vi "Keithley617_IV.vi"() -> ()   [LabVIEW 2015, in "Keithley617.lvlib"]
uses:
  Keithley617.lvlib
  Keithley617_GPIB_Commands.ctl
panel:
  in  "Array":T1(array[cluster])
  out "IV- Live Plot":cluster{"X":dbl, "Y":dbl}[](graph)
  out "Error Out":errorcluster
  in  "Error In":errorcluster
  in  "GPIB Address String":string="27"
  in  "Input Parameters":T2={"Start Voltage"=0.0, "End Voltage"=0.0, "Voltage Step"=0.0, "Step Time (ms)"=100.0}
  out "IV-result":cluster{"X":dbl, "Y":dbl}[](graph)
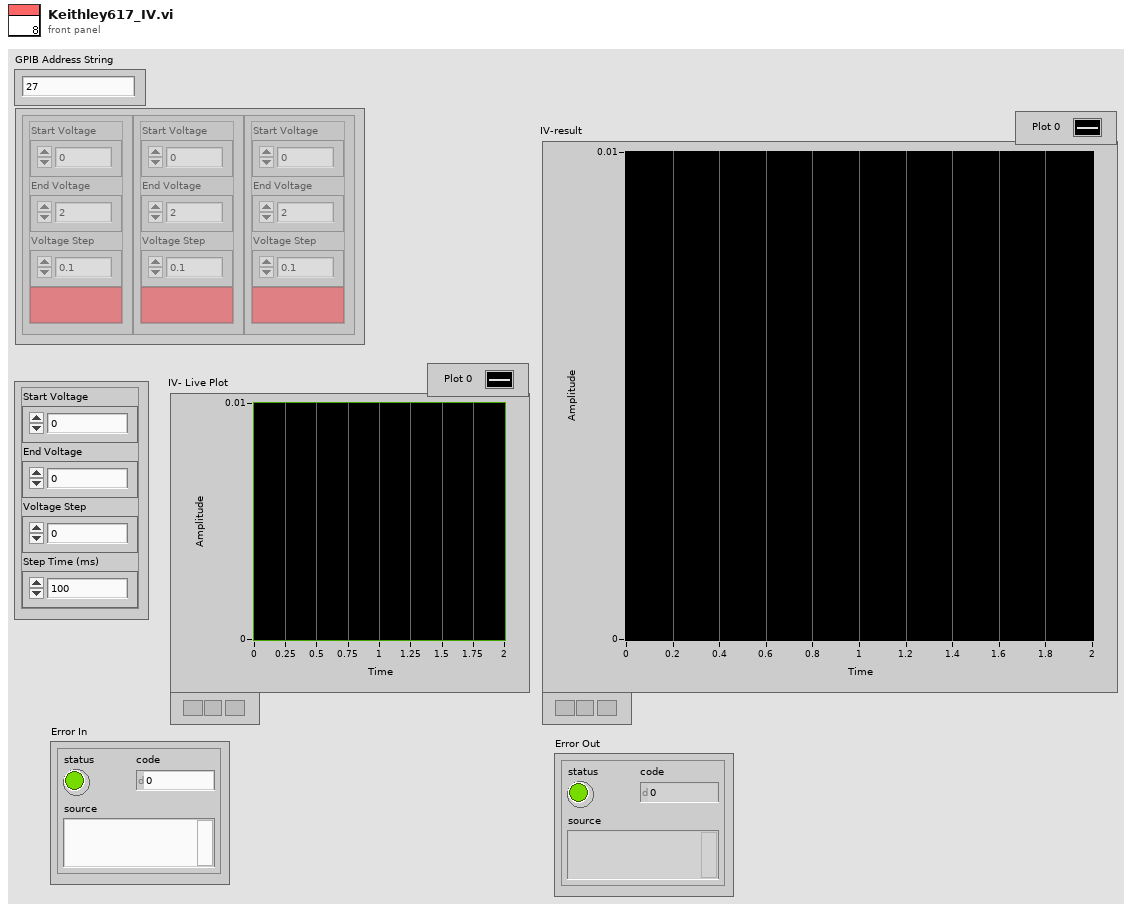
[diagram p1: front panel]
types:
  T1 = cluster{"Start Voltage":dbl, "End Voltage":dbl, "Voltage Step":dbl, "Enable?":bool}[]
  T2 = cluster{"Start Voltage":dbl, "End Voltage":dbl, "Voltage Step":dbl, "Step Time (ms)":dbl}
  T3 = typedef "Keithley617_GPIB_Commands.ctl" = string
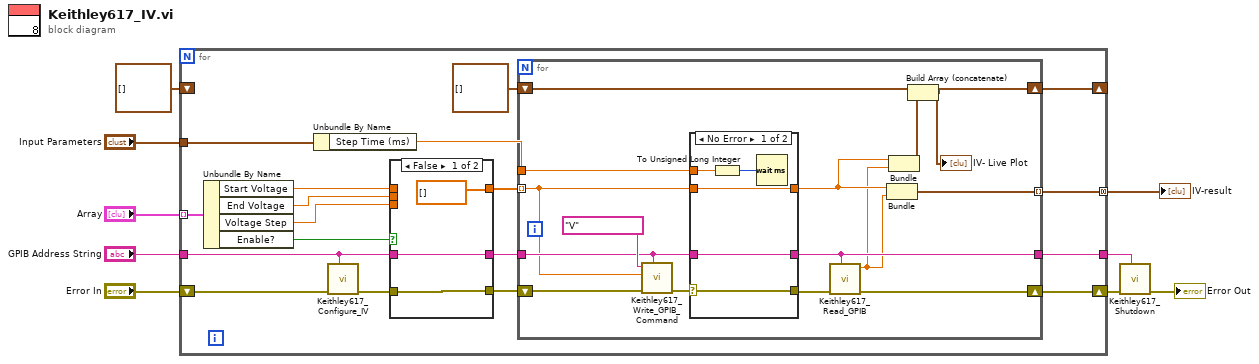
[diagram p0: block diagram]
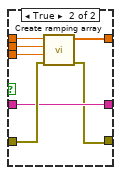
[diagram p2: hidden frame]
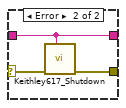
[diagram p3: hidden frame]
diagram:
  n1 = for {
    tunnel: "Input Parameters" -> [w24]
    tunnel: "Array" -> [w19] mode=indexing
    tunnel: [w22] -> w6 mode=concatenating
    tunnel: "GPIB Address String" -> [w10]
    tunnel: [w21] -> w3
    shift-right: [w17] -> _
    shift-left: cluster{"Numeric":dbl, "Output value":dbl}[] [] -> [_]
    shift-right: [w13] -> w5
    shift-left: "Error In" -> [w11]
    n2 = Unbundle By Name(w19) -> ("Start Voltage"=w27:dbl, "End Voltage"=w20:dbl, "Voltage Step"=w26:dbl, "Enable?"=w18:bool)
    n3 = Unbundle By Name(w24) -> ("Step Time (ms)"=w23:dbl)
    n4 = call "Keithley617_Configure_IV.vi"("GPIB Address String"=w10, "Error In"=w11) -> ("Error Out"=w12:errorcluster)  [unwired: 9 in]
    n5 = case shown="False" w18 {
      tunnel: w27 -> [_ w37]
      tunnel: w26 -> [_ w36]
      tunnel: [dbl[] [] w35] -> w25
      tunnel: w12 -> [w29 w34]
      tunnel: [w29 w31] -> w14
      tunnel: w20 -> [_ w33]
      tunnel: [w30 w32] -> w15
      tunnel: w10 -> [w30 w32]
      frame False {
      }
      frame True {
        n6 = call "Create ramping array.vi"("Error In"=w34, "Delta"=w36, "End"=w33, "Start"=w37) -> ("Error Out"=w31:errorcluster, "Output Array (1D)"=w35:dbl[])  [unwired: 5 in, 1 out]
      }
    }
    n7 = for {
      tunnel: w25 -> [w46] mode=indexing
      tunnel: w23 -> [w50]
      tunnel: w15 -> [w48]
      tunnel: [w45] -> w22 mode=indexing
      tunnel: [w43] -> w21
      shift-right: [w41] -> w17
      shift-left: cluster{"Numeric":dbl, "Output value":dbl}[] [] -> [w39]
      shift-right: [w44] -> w13
      shift-left: w14 -> [w52]
      n8 = call "Keithley617_Write_GPIB_Command.vi"("GPIB Address String"=w48, "Error In"=w52, "Value"=w46, "Command"=T3 "V") -> ("Error Out"=w51:errorcluster)  [unwired: 7 in]
      n9 = case shown="No Error" w51 {
        selector: w51 -> [w55 w60]
        tunnel: w50 -> [w57 _]
        tunnel: [w55 w59] -> w47
        tunnel: w48 -> [w54 w58]
        tunnel: [w54 w58] -> w43
        tunnel: w46 -> [w53 _]
        tunnel: [w53 _] -> w42
        frame No Error {
          n10 = To Unsigned Long Integer(number=w57) -> (unsigned 32bit integer=w56:u32)
          n11 = Wait (ms)(milliseconds to wait=w56) -> ()  [unwired: 1 out]
        }
        frame Error {
          n12 = call "Keithley617_Shutdown.vi"("GPIB Address String"=w58, "Error In"=w60) -> ("Error Out"=w59:errorcluster)  [unwired: 9 in]
        }
      }
      n13 = call "Keithley617_Read_GPIB.vi"("GPIB Address String"=w43, "Error In"=w47) -> ("Error Out"=w44:errorcluster, "Output value"=w38:dbl)  [unwired: 8 in]
      n14 = Bundle("Numeric"=w42, "Output value"=w38) -> (w45:cluster{"Numeric":dbl, "Output value":dbl})  [unwired: 1 in]
      n15 = Bundle("Numeric"=w42, "Output value"=w38) -> (w40:cluster{"Numeric":dbl, "Output value":dbl})  [unwired: 1 in]
      n16 = Build Array (concatenate)(w39, w40) -> (w41:cluster{"Numeric":dbl, "Output value":dbl}[])
      "IV- Live Plot" <- w41
    }
  }
  "IV-result" <- w6
  n17 = call "Keithley617_Shutdown.vi"("GPIB Address String"=w3, "Error In"=w5) -> ("Error Out"=→"Error Out":errorcluster)  [unwired: 9 in]
